vi "eventListenerTest.vi"() -> ()   [LabVIEW 2020]
uses:
  Global stop DAQ.vi
  Global stop.vi
panel:
  out "Numeric":i32
  in  "Milliseconds to wait":u32
  in  "lines":tag
  out "Label.Text":string
  out "Class Name":string
  in  "stop":bool
  in  "Media Stop Button":bool
  in  "Play Button":bool
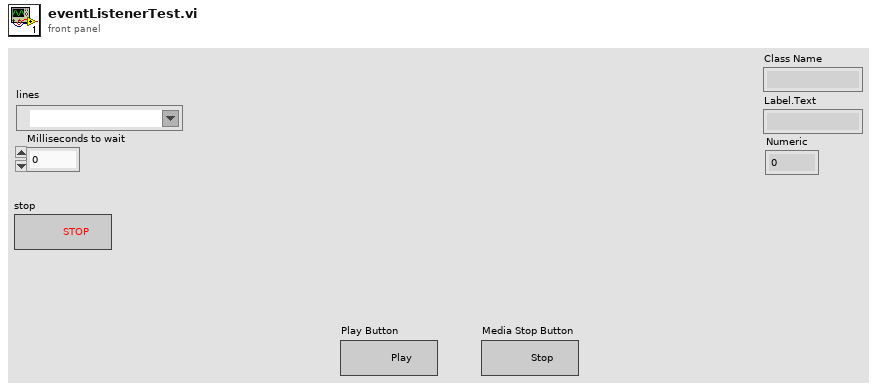
[diagram p1: front panel]
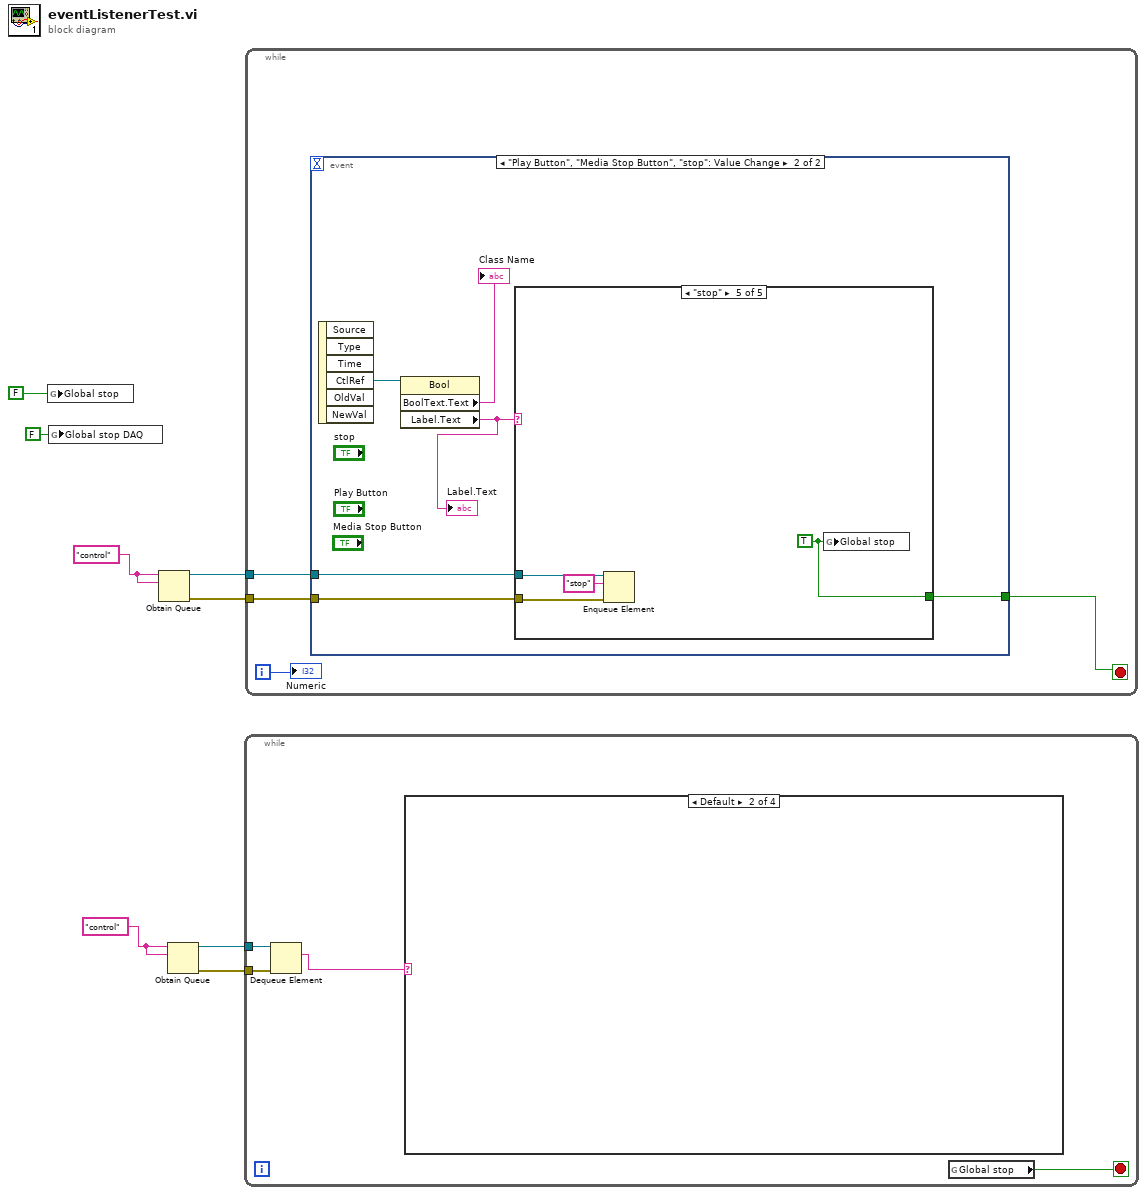
[diagram p0: block diagram]
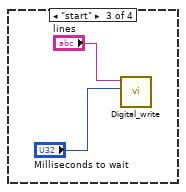
[diagram p3: hidden frame]
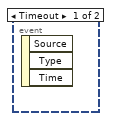
[diagram p5: hidden frame]
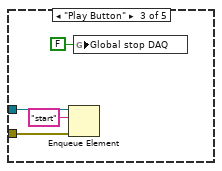
[diagram p8: hidden frame]
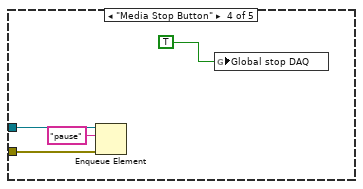
[diagram p9: hidden frame]
diagram:
  w5 = "control" ("name (unnamed)")
  w6 = "control" ("name (unnamed)")
  n1 = global write "Global stop.vi" "Global stop"(FALSE) -> ()
  n2 = global write "Global stop DAQ.vi" "Global stop DAQ"(FALSE) -> ()
  n3 = Obtain Queue(name (unnamed)=w6, element data type=w6) -> (queue out=w8:refnum<queue>, error out=w7:errorcluster)  [unwired: 3 in, 1 out]
  n4 = Obtain Queue(name (unnamed)=w5, element data type=w5) -> (queue out=w4:refnum<queue>, error out=w3:errorcluster)  [unwired: 3 in, 1 out]
  n5 = while {
    tunnel: w4 -> [w12]
    tunnel: w3 -> [w11]
    stop <- w9 stop-if-true
    n6 = Dequeue Element(queue=w12, error in (no error)=w11) -> (element=w10:string)  [unwired: 1 in, 3 out]
    n7 = case shown="Default" w10 {
      frame "pause" {
      }
      frame Default {
      }
      frame "start" {
        n8 = call "Digital_write.vi"("Milliseconds to wait"="Milliseconds to wait", "lines"="lines") -> ()  [unwired: 10 in]
      }
      frame "stop" {
      }
    }
    n9 = global read "Global stop.vi" "Global stop"() -> (w9:bool)
  }
  n10 = while {
    tunnel: w8 -> [w18]
    tunnel: w7 -> [w17]
    i -> [w16]
    stop <- w15 stop-if-true
    n11 = event shown="[1] \"Play Button\", \"Media Stop Button\", \"stop\": Value Change" {
      selector: _ -> [_ _]
      dyn-events: _ -> [_ _]
      timeout: _ -> [_ _]
      tunnel: w18 -> [_ w21]
      tunnel: w17 -> [_ w20]
      tunnel: [_ w19] -> w15
      event Timeout {
        n12 = event-data() -> ()  [unwired: 1 in, 3 out]
      }
      event "Play Button", "Media Stop Button", "stop": Value Change {
        n13 = event-data() -> ("CtlRef"=w24:refnum<vi>)  [unwired: 1 in, 5 out]
        n14 = property class="Bool"(reference=w24) -> ("BoolText.Text"=→"Class Name":string, "Label.Text"=w22:string)  [unwired: 1 in, 2 out]
        "Label.Text" <- w22
        n15 = case shown="\"stop\"" w22 {
          tunnel: w21 -> [_ _ w28 w31 w35]
          tunnel: w20 -> [_ _ w27 w30 w34]
          tunnel: [_ _ _ _ w33] -> w19
          frame "False", Default {
          }
          frame "True" {
          }
          frame "Play Button" {
            n16 = Enqueue Element(queue=w28, element="start", error in (no error)=w27) -> ()  [unwired: 1 in, 3 out]
            n17 = global write "Global stop DAQ.vi" "Global stop DAQ"(FALSE) -> ()
          }
          frame "Media Stop Button" {
            n18 = Enqueue Element(queue=w31, element="pause", error in (no error)=w30) -> ()  [unwired: 1 in, 3 out]
            n19 = global write "Global stop DAQ.vi" "Global stop DAQ"(TRUE) -> ()
          }
          frame "stop" {
            w33 = TRUE
            n20 = Enqueue Element(queue=w35, element="stop", error in (no error)=w34) -> ()  [unwired: 1 in, 3 out]
            n21 = global write "Global stop.vi" "Global stop"(w33) -> ()
          }
        }
      }
    }
    "Numeric" <- w16
  }
